vi "Initialize.vi"(0 "NIPKG_LV in":refnum<class "NIPKG_LV.lvclass">) -> (4 "NIPKG_LV out":refnum<class "NIPKG_LV.lvclass">)   [LabVIEW 2017, in "CL_G3_VIComponentBuilder.lvlib" / "NIPKG_LV.lvclass"]
doc: "Calculates the build machine folder path for the committ behavior based on the export's defintion."
uses:
  NIPKG_LV.lvclass
  C:/builds/Component BuilderBT/SrcDist/Exports/Exports/Export.lvclass
  Commit Behavior/CommitNIPKG_LV/CommitNIPKG_LV.lvclass
  C:/builds/Component BuilderBT/SrcDist/Commit Behavior/Commit/Commit.lvclass
  Exports/Export.lvclass/Export.ctl
  NIPKG_LV.lvclass/NIPKG_LV.ctl
  Exports/Accessors/Read Commit behavior.vi
  Accessors/Read Build Machine Feed Folderpath.vi
  Exports/Accessors/Write Commit behavior.vi
  Exports/Accessors/Write Export Operation Errors.vi
  NI Build Specification_LV/NI Build Specification_LV.lvclass
  Commit Behavior/Commit/Commit.lvclass
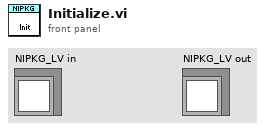
[diagram p1: front panel]
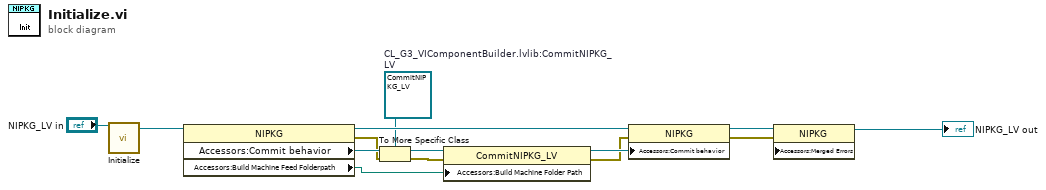
[diagram p0: block diagram]
diagram:
  w9 = refnum<class "CommitNIPKG_LV.lvclass"> refnum  # CL_G3_VIComponentBuilder.lvlib:CommitNIPKG_LV
  n1 = call-parent "Initialize.vi"("NI Build Specification_LV in"="NIPKG_LV in") -> ("NI Build Specification_LV out"=w13:refnum<class "NIPKG_LV.lvclass">)  [unwired: 14 in]
  n2 = property class="NIPKG"(reference=w13) -> (reference out=w12:refnum<class "NIPKG_LV.lvclass">, error out=w5:errorcluster, "Accessors:Commit behavior"=w11:refnum<class "Commit.lvclass">, "Accessors:Build Machine Feed Folderpath"=w8:path)  [unwired: 1 in]
  n3 = To More Specific Class(target class=w9, reference=w11, error in=w5) -> (specific class reference=w10:refnum<class "CommitNIPKG_LV.lvclass">, error out=w4:errorcluster)
  n4 = property class="CommitNIPKG_LV"(reference=w10, error in=w4, "Accessors:Build Machine Folder Path"=w8) -> (reference out=w6:refnum<class "CommitNIPKG_LV.lvclass">, error out=w3:errorcluster)
  n5 = property class="NIPKG"(reference=w12, error in=w3, "Accessors:Commit behavior"=w6) -> (reference out=w7:refnum<class "NIPKG_LV.lvclass">, error out=w1:errorcluster)
  n6 = property class="NIPKG"(reference=w7, "Accessors:Merged Errors"=w1) -> (reference out=→"NIPKG_LV out":refnum<class "NIPKG_LV.lvclass">)  [unwired: 1 in, 1 out]
